vi "SigInfo SaveMZInfo.vi"(7 "Function":T1=enum."Set SigInfo", 8 "error in (no error)":errorcluster, 10 "SigInfo":T3, 11 "Signal Remarks input":T2) -> (0 "error out":errorcluster, 3 "Signal Remarks output":T2, 5 "ID":u64=3617166582204)   [LabVIEW 2018, in "SigInfo.lvclass"]
uses:
  SigInfo.lvclass
  SigInfo.ctl
  SigInfo.lvclass/SigInfo.ctl
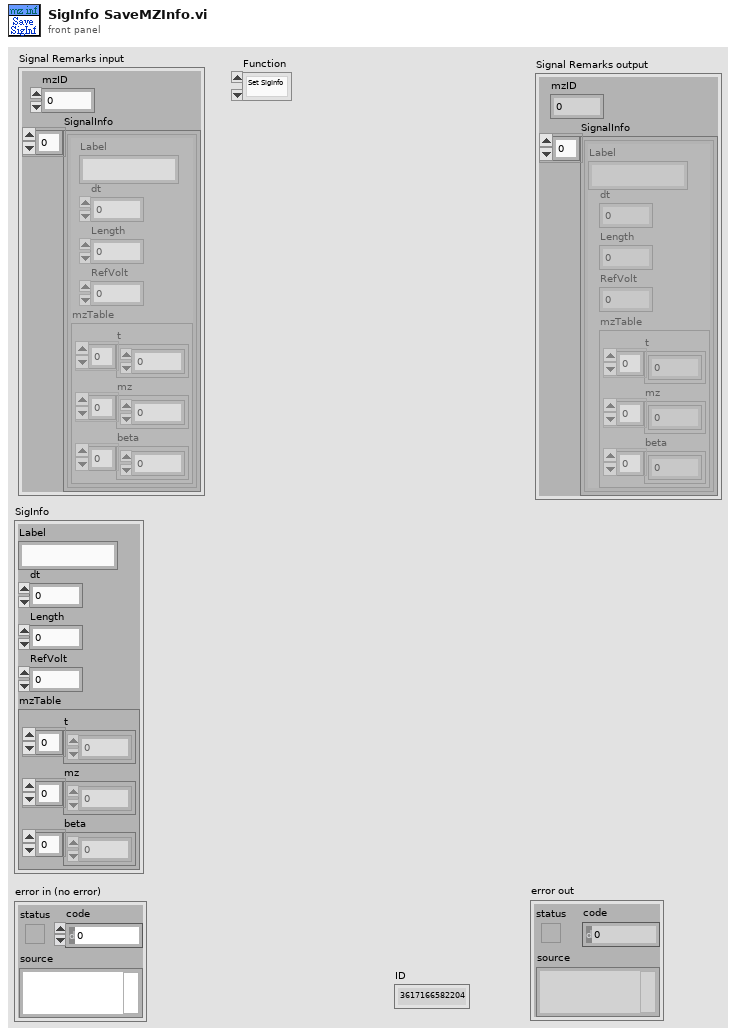
[diagram p1: front panel]
types:
  T1 = typedef "SigInfo.ctl" = enum16{"New mzList", "Set SigInfo", "Get SigInfo", "Append", "End"}
  T2 = cluster{"mzID":u64, "SignalInfo":cluster{"Label":string, "dt":dbl, "Length":u32, "RefVolt":dbl, "mzTable":cluster{"t":dbl[], "mz":dbl[], "beta":dbl[]}}[]}
  T3 = cluster{"Label":string, "dt":dbl, "Length":u32, "RefVolt":dbl, "mzTable":cluster{"t":dbl[], "mz":dbl[], "beta":dbl[]}}
  T4 = enum16{"open", "replace", "create", "open or create", "replace or create", "replace or create with confirmation"}
  T5 = typedef "Semaphore RefNum" = refnum<k1>
  T6 = cluster{"Label":string, "dt":dbl, "Length":u32, "RefVolt":dbl, "mzTable":cluster{"t":dbl[], "mz":dbl[], "beta":dbl[]}}[]
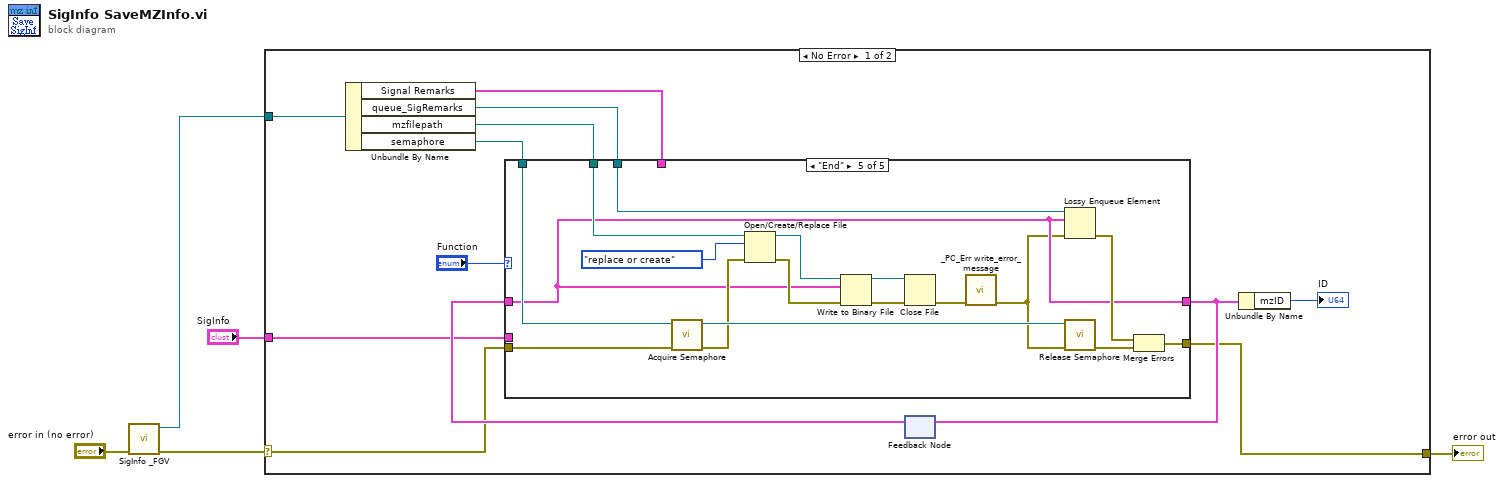
[diagram p0: block diagram]
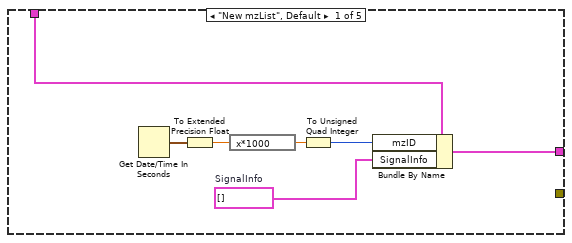
[diagram p2: hidden frame]
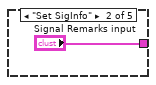
[diagram p3: hidden frame]
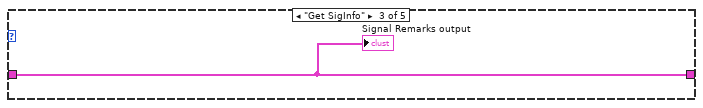
[diagram p4: hidden frame]
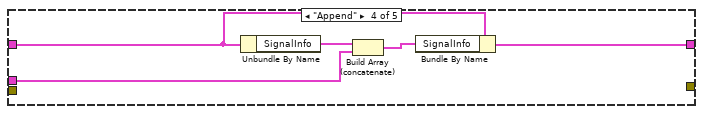
[diagram p5: hidden frame]
diagram:
  n1 = call "SigInfo _FGV.vi"("error in (no error)"="error in (no error)") -> ("error out"=w3:errorcluster, "mzInfo out"=w2:refnum<class "SigInfo.lvclass">)  [unwired: 9 in]
  n2 = case shown="No Error" w3 {
    selector: w3 -> [w7 w49]
    tunnel: [w6 w49] -> w5
    tunnel: w2 -> [w17 _]
    tunnel: "SigInfo" -> [w9 _]
    frame No Error {
      n3 = Unbundle By Name(w17) -> ("Signal Remarks"=w15:T2, "queue_SigRemarks"=w16:refnum<queue>, "mzfilepath"=w13:path, "semaphore"=w12:T5)
      n4 = feedback #1() -> (w14:T2)  [unwired: 1 in]
      n5 = case shown="\"End\"" "Function" {
        tunnel: w16 -> [_ _ _ _ w48]
        tunnel: w9 -> [_ _ _ w27 _]
        tunnel: w15 -> [w22 _ _ _ _]
        tunnel: [w21 "Signal Remarks input" w26 w28 w34] -> w11
        tunnel: w14 -> [_ _ w26 w29 w34]
        tunnel: w13 -> [_ _ _ _ w45]
        tunnel: w12 -> [_ _ _ _ w44]
        tunnel: w7 -> [_ _ _ _ w38]
        tunnel: [_ _ _ _ w35] -> w6
        frame "New mzList", Default {
          w18 = T6 []  # SignalInfo
          n6 = Get Date/Time In Seconds() -> (seconds since 1Jan1904=w24:timestamp)
          n7 = To Extended Precision Float(1:w24) -> (0:w23:ext)
          n8 = expression code="x*1000"(w23) -> (w20:ext)
          n9 = To Unsigned Quad Integer(1:w20) -> (0:w19:u64)
          n10 = Bundle By Name(cluster=w22, "mzID"=w19, "SignalInfo"=w18) -> (w21:T2)
        }
        frame "Set SigInfo" {
        }
        frame "Get SigInfo" {
          "Signal Remarks output" <- w26
        }
        frame "Append" {
          n11 = Unbundle By Name(w29) -> ("SignalInfo"=w31:T6)
          n12 = Build Array (concatenate)(w31, w27) -> (w30:T6)
          n13 = Bundle By Name(cluster=w29, "SignalInfo"=w30) -> (w28:T2)
        }
        frame "End" {
          n14 = call <vilib>:"Acquire Semaphore.vi"("error in (no error)"=w38, "semaphore"=w44) -> ("error out"=w42:errorcluster, "semaphore out"=w43:T5)  [unwired: 3 in, 1 out]
          n15 = Open/Create/Replace File(file path (use dialog)=w45, error in=w42, operation (0:open)=T4."replace or create") -> (refnum out=w40:refnum<file>, error out=w39:errorcluster)  [unwired: 3 in, 1 out]
          n16 = Write to Binary File(file (use dialog)=w40, data=w34, error in=w39) -> (refnum out=w46:refnum<file>, error out=w47:errorcluster)  [unwired: 3 in, 1 out]
          n17 = Close File(refnum=w46, error in=w47) -> (error out=w33:errorcluster)  [unwired: 1 out]
          n18 = call "_PC_Err write_error_message.vi"("error in"=w33) -> ("error out"=w32:errorcluster)  [unwired: 10 in]
          n19 = Lossy Enqueue Element(queue=w48, element=w34, error in (no error)=w32) -> (error out=w36:errorcluster)  [unwired: 3 out]
          n20 = call <vilib>:"Release Semaphore.vi"("error in (no error)"=w32, "semaphore"=w43) -> ("error out"=w37:errorcluster)  [unwired: 4 in, 1 out]
          n21 = Merge Errors(w36, w37) -> (w35:errorcluster)
        }
      }
      n22 = feedback-in #1(w11) -> ()
      n23 = Unbundle By Name(w11) -> ("mzID"=→"ID":u64)
    }
    frame Error {
    }
  }
  "error out" <- w5
